vi "Remove Multiple Wheels from Steering Frame.vi"(8 "error in (no error)":errorcluster, 10 "wheel indexes":i32[](array[numeric]), 11 "steering frame in":refnum<class "NI_Robotics_Steering Frame.lvclass">) -> (0 "error out":errorcluster, 1 "found?":bool[](array[boolean]), 2 "removed wheels":refnum<class "NI_Robotics_Wheel.lvclass">[](array[class]), 3 "steering frame out":refnum<class "NI_Robotics_Steering Frame.lvclass">, 4 "frame angles (rad)":dbl[](array[numeric]), 5 "y positions":dbl[](array[numeric]), 7 "x positions":dbl[](array[numeric]))   [LabVIEW 2017, in "NI_Robotics_Steering Frame.lvclass"]
doc: "Removes the wheel or wheels you specify from <B>steering frame in</B>. You must manually select the polymorphic instance to use."
uses:
  <vilib>/robotics/Steering/Steering Frame/NI_Robotics_Steering Frame.lvclass
  <vilib>/robotics/Steering/Wheel/NI_Robotics_Wheel.lvclass
  <vilib>/robotics/Steering/Steering Frame/NI_Robotics_Steering Frame.lvclass/NI_Robotics_Steering Frame.ctl
  <vilib>/robotics/Utilities/NI_Robotics Utilities.lvlib
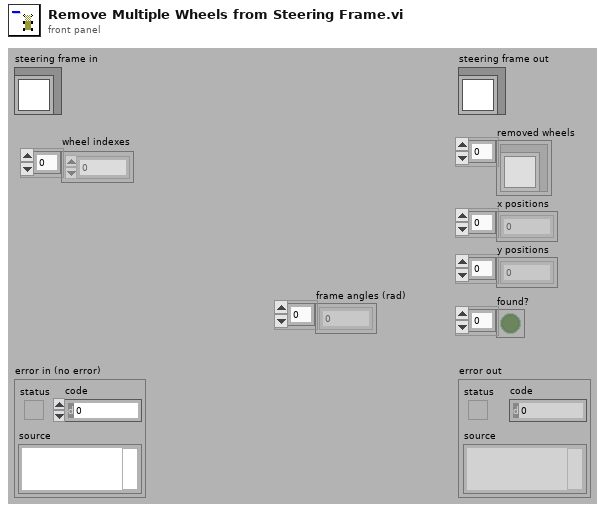
[diagram p1: front panel]
types:
  T1 = typedef "NI_Robotics_Steering Frame.lvclass/Wheel Orientation.ctl" = cluster{"wheel":refnum<class "NI_Robotics_Wheel.lvclass">, "x position":dbl, "y position":dbl, "frame angle (rad)":dbl}
  T2 = typedef "NI_Robotics_Wheel.lvclass/Wheel State.ctl" = cluster{"wheel name":string, "forward angular velocity":dbl, "caster angular velocity":dbl, "caster wheel angle (rad)":dbl, "steering angle (rad)":dbl}
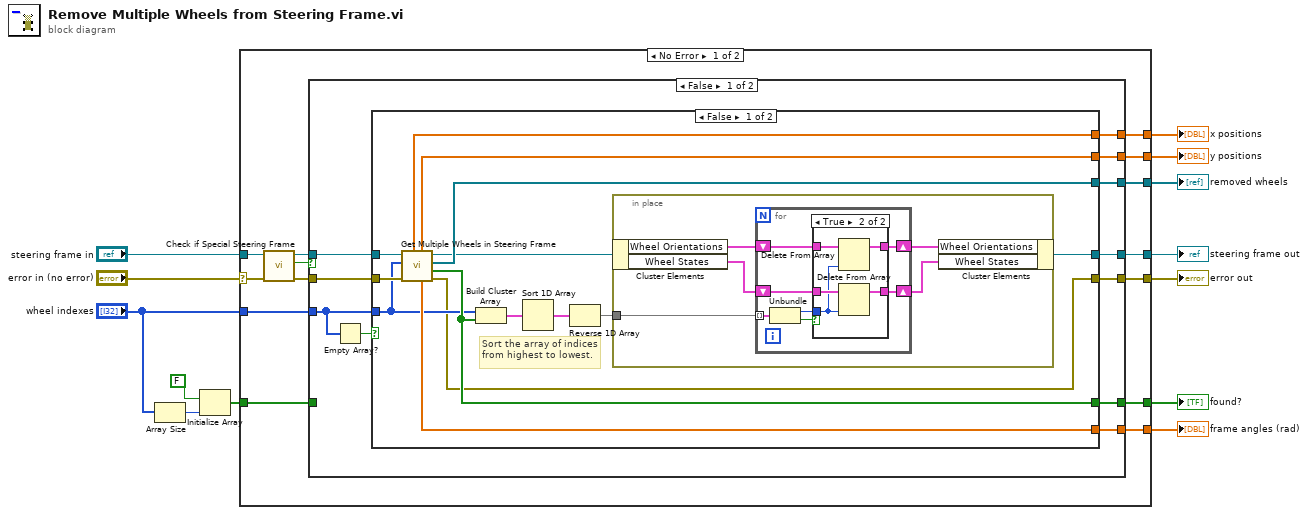
[diagram p0: block diagram]
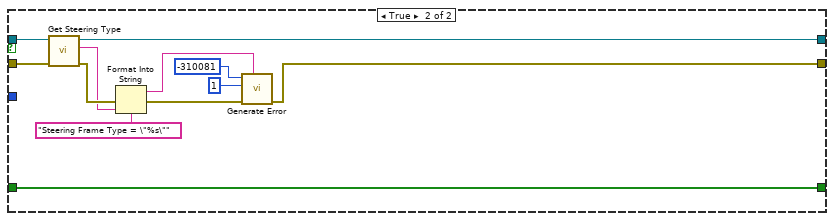
[diagram p4: hidden frame]
diagram:
  n1 = Array Size(array="wheel indexes") -> (size(s)=w2:i32)
  n2 = Initialize Array(FALSE, w2) -> (w1:bool[])
  n3 = case shown="No Error" "error in (no error)" {
    selector: "error in (no error)" -> [w23 w88]
    tunnel: [w20 w88] -> w12
    tunnel: [w27 w87] -> w10
    tunnel: "steering frame in" -> [w25 w87]
    tunnel: "wheel indexes" -> [w26 _]
    tunnel: [w19 _] -> w9
    tunnel: [w18 _] -> w8
    tunnel: [w17 _] -> w7
    tunnel: [w16 _] -> w6
    tunnel: [w15 w86] -> w5
    tunnel: w1 -> [w14 w86]
    frame No Error {
      n4 = call-dynamic "Check if Special Steering Frame.vi"("error in (no error)"=w23, "steering frame in"=w25) -> ("error out"=w21:errorcluster, "special?"=w22:bool, "steering frame out"=w24:refnum<class "NI_Robotics_Steering Frame.lvclass">)  [unwired: 7 in]
      n5 = case shown="False" w22 {
        tunnel: [w36 w77] -> w27
        tunnel: w26 -> [w29 _]
        tunnel: w24 -> [w38 w78]
        tunnel: w21 -> [w35 w76]
        tunnel: [w34 w85] -> w20
        tunnel: [w33 _] -> w19
        tunnel: [w30 _] -> w18
        tunnel: [w31 _] -> w17
        tunnel: [w32 _] -> w16
        tunnel: [w28 w82] -> w15
        tunnel: w14 -> [_ w82]
        frame False {
          n6 = Empty Array?(array=w29) -> (empty?=w37:bool)
          n7 = case shown="False" w37 {
            tunnel: w38 -> [w52 w72]
            tunnel: w35 -> [w51 w73]
            tunnel: [w39 w72] -> w36
            tunnel: [w40 w73] -> w34
            tunnel: [w50 _] -> w33
            tunnel: [w49 _] -> w32
            tunnel: [w48 _] -> w31
            tunnel: [w47 _] -> w30
            tunnel: w29 -> [w42 _]
            tunnel: [w43 _] -> w28
            frame False {
              # "Sort the array of indices from highest to lowest."
              n8 = call <vilib>:"Get Multiple Wheels in Steering Frame.vi"("error in (no error)"=w51, "wheel indexes"=w42, "steering frame in"=w52) -> ("error out"=w40:errorcluster, "found?"=w43:bool[], "wheels"=w50:refnum<class "NI_Robotics_Wheel.lvclass">[], "steering frame out"=w45:refnum<class "NI_Robotics_Steering Frame.lvclass">, "frame angles (rad)"=w49:dbl[], "y positions"=w48:dbl[], "x positions"=w47:dbl[])  [unwired: 2 in]
              n9 = Build Cluster Array(w42, w43) -> (w41:cluster{"Numeric":i32, bool}[])
              n10 = Sort 1D Array(array=w41) -> (sorted array=w46:cluster{"Numeric":i32, bool}[])
              n11 = Reverse 1D Array(array=w46) -> (reversed array=w44:cluster{"Numeric":i32, bool}[])
              n12 = in-place {
                in-place-border: w44 -> [w57]
                n13 = in-place-cluster #1(w45) -> ("Wheel Orientations"=w56:T1[], "Wheel States"=w54:T2[])
                n14 = for {
                  tunnel: w57 -> [w62] mode=indexing
                  shift-right: [w63] -> w55
                  shift-left: w56 -> [w64]
                  shift-right: [w58] -> w53
                  shift-left: w54 -> [w59]
                  n15 = Unbundle(w62) -> ("Numeric"=w60:i32, w61:bool)
                  n16 = case shown="True" w61 {
                    tunnel: w64 -> [w66 w71]
                    tunnel: w60 -> [_ w68]
                    tunnel: [w66 w70] -> w63
                    tunnel: w59 -> [w65 w69]
                    tunnel: [w65 w67] -> w58
                    frame False {
                    }
                    frame True {
                      n17 = Delete From Array(array=w71, index=w68) -> (array with subset deleted=w70:T1[])  [unwired: 1 in, 1 out]
                      n18 = Delete From Array(array=w69, index=w68) -> (array with subset deleted=w67:T2[])  [unwired: 1 in, 1 out]
                    }
                  }
                }
                n19 = in-place-cluster #1("Wheel Orientations"=w55, "Wheel States"=w53) -> (w39:refnum<class "NI_Robotics_Steering Frame.lvclass">)
              }
            }
            frame True {
            }
          }
        }
        frame True {
          n20 = call-dynamic "Get Steering Type.vi"("error in (no error)"=w76, "steering frame in"=w78) -> ("error out"=w81:errorcluster, "steering type"=w80:string, "steering frame out"=w77:refnum<class "NI_Robotics_Steering Frame.lvclass">)  [unwired: 7 in]
          n21 = Format Into String(format string="Steering Frame Type = \"%s\"", error in=w81, w80) -> (resulting string=w75:string, error out=w74:errorcluster)  [unwired: 1 in]
          n22 = call <vilib>:"Generate Error.vi"("<append> (\"\")"=w75, "error in (no error)"=w74, "chain levels to remove (1)"=1, "code"=-310081) -> ("error out"=w85:errorcluster)  [unwired: 7 in]
        }
      }
    }
    frame Error {
    }
  }
  "error out" <- w12
  "steering frame out" <- w10
  "removed wheels" <- w9
  "x positions" <- w8
  "y positions" <- w7
  "frame angles (rad)" <- w6
  "found?" <- w5
